vi "dashboard_vision_processing.vi"(11 "Image Ctl":refnum<vi>) -> ()   [LabVIEW 2011]
uses:
  dashboard_return_data.ctl
  2012vision/Camera State.ctl
  <vilib>/vision/NI_Vision_Development_Module.lvlib
panel:
  out "error out":errorcluster
  in  "Threshold Range":cluster{"Lower value":sgl, "Upper value":sgl}={"Lower value"=217.0, "Upper value"=255.0} {"Upper value" format="%.2f"; "Lower value" format="%.2f"}
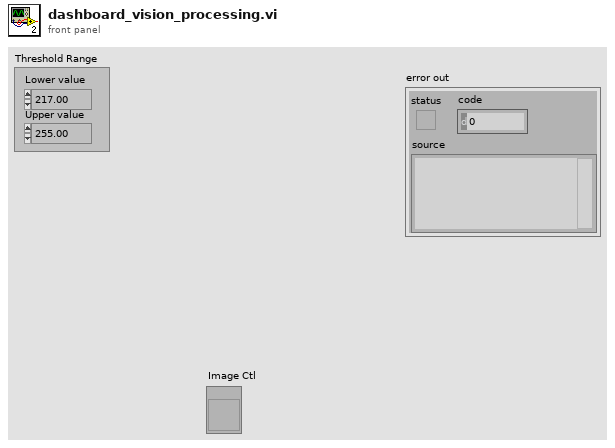
[diagram p1: front panel]
types:
  T1 = typedef "Image Type" = u32
  T2 = typedef "IMAQ Image.ctl" = refnum<image>
  T3 = typedef "dashboard_return_data.ctl" = cluster{"Targetting Output":cluster{"X Position":dbl, "Distance":dbl, "Camera State":T4}, "Camera Error Status":errorcluster, "packet send timestamp":u32, "img process timestamp":u32}
  T4 = typedef "Camera State.ctl" = enum16{"No Targets", "Low Confidence", "Medium Confidence", "High Confidence", "Camera Error"}
  T5 = enum32{"AutoM", "Close", "Dilate", "Erode", "Gradient", "Gradient in", "Gradient out", "HitMiss", "Open", "PClose", "POpen", "Thick", "Thin"}
  T6 = cluster{"Rect Coverage":dbl, "Aspect Ratio":dbl, "X Edge Strength":dbl, "Y Edge Strength":dbl}
  T7 = typedef "WPI_CameraImageSize.ctl" = enum16{"640x480", "320x240", "160x120"}
  T8 = cluster{"fps dashboard":i32, "compression dashboard":i32, "img size dashboard":T7}
  T9 = cluster{cluster{"Left":dbl, "Top":dbl, "Right":dbl, "Bottom":dbl}, cluster{"Score":dbl, "Score":dbl, "X Score":dbl, "Y Score":dbl}, "Clipped Edge":cluster{"Left":bool, "Top":bool, "Right":bool, "Bottom":bool}}[]
  T10 = cluster{"X Position":dbl, "Distance":dbl, "Camera State":T4}
  T11 = typedef "Diamond Target Output.ctl" = cluster{"Position":cluster{"X":dbl, "Y":dbl, "Distance":dbl}, "Est. Position":T12, "Target Confidence":T13}
  T12 = typedef "Rectangle Position.ctl" = enum16{"Unknown", "Top", "Right", "Left", "Bottom"}
  T13 = typedef "Target Confidence.ctl" = enum16{"Good", "Good-Clipped Y", "Marginal-Clipped X"}
  T14 = typedef "Line.ctl" = cluster{"First Point":cluster{"X":dbl, "Y":dbl, "Index":dbl}, "Second Point":cluster{"X":dbl, "Y":dbl, "Index":dbl}, "theta":dbl, "Direction":T15, "Line Confidence":T16}
  T15 = typedef "Direction.ctl" = enum16{"Rt", "Rt-Up", "Up", "Lt-Up", "Lt", "Lt-Dn", "Dn", "Rt-Dn", "Unknown"}
  T16 = typedef "Line Confidence.ctl" = enum16{"Good", "Bad"}
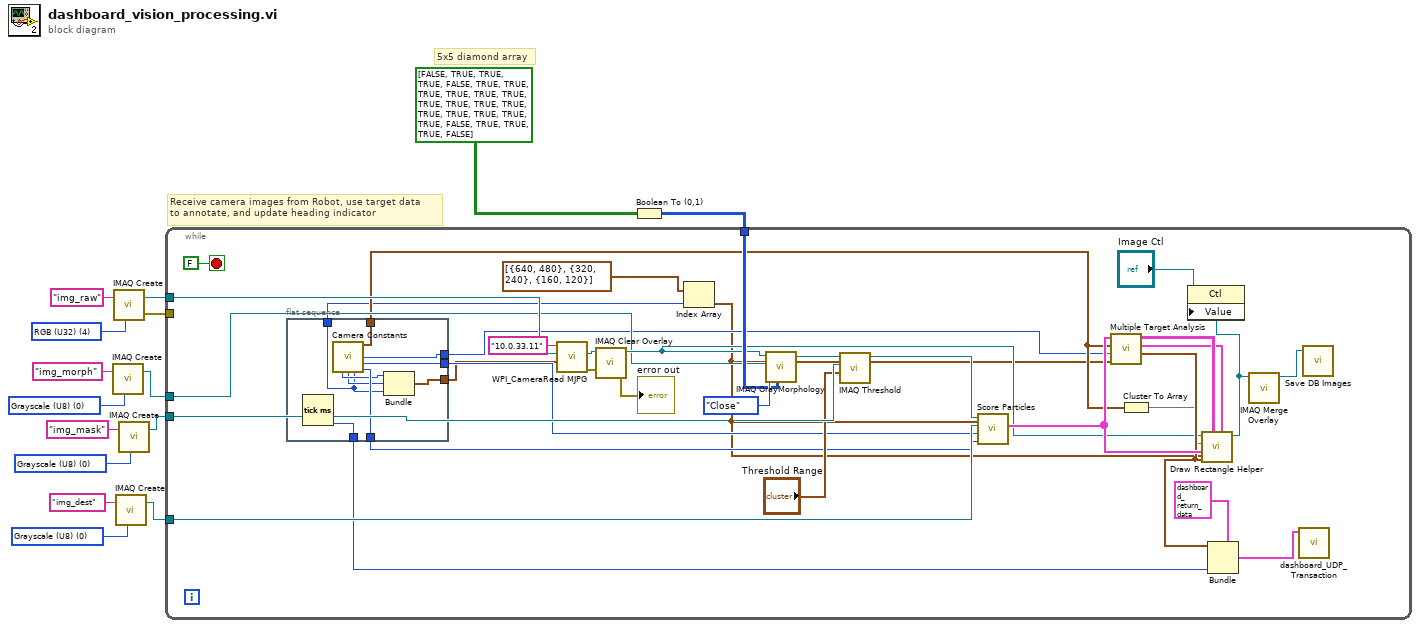
[diagram p0: block diagram]
diagram:
  w4 = T1 0 items=["Grayscale (U8)", "Grayscale (I16)", "Grayscale (SGL)", "Complex (CSG)", "RGB (U32)", "HSL (U32)", "RGB (U64)"] ("Image Type")
  w14 = T1 0 items=["Grayscale (U8)", "Grayscale (I16)", "Grayscale (SGL)", "Complex (CSG)", "RGB (U32)", "HSL (U32)", "RGB (U64)"] ("Image Type")
  w11 = T1 0 items=["Grayscale (U8)", "Grayscale (I16)", "Grayscale (SGL)", "Complex (CSG)", "RGB (U32)", "HSL (U32)", "RGB (U64)"] ("Image Type")
  w7 = T1 4 items=["Grayscale (U8)", "Grayscale (I16)", "Grayscale (SGL)", "Complex (CSG)", "RGB (U32)", "HSL (U32)", "RGB (U64)"] ("Image Type")
  # "5x5 diamond array"
  # "Receive camera images from Robot, use target data\nto annotate, and update heading indicator"
  n1 = call "IMAQ Create"("Image Name"="img_morph", "Image Type"=w11) -> ("New Image"=w13:T2)  [unwired: 2 in, 2 out]
  n2 = call "IMAQ Create"("Image Name"="img_raw", "Image Type"=w7) -> ("New Image"=w9:T2, "error out"=w10:errorcluster)  [unwired: 2 in, 1 out]
  n3 = call "IMAQ Create"("Image Name"="img_dest", "Image Type"=w4) -> ("New Image"=w3:T2)  [unwired: 2 in, 2 out]
  n4 = call "IMAQ Create"("Image Name"="img_mask", "Image Type"=w14) -> ("New Image"=w6:T2)  [unwired: 2 in, 2 out]
  n5 = Boolean To (0,1)(Boolean=bool[][] [[FALSE, TRUE, TRUE, TRUE, FALSE], [TRUE, TRUE, TRUE, TRUE, TRUE], [TRUE, TRUE, TRUE, TRUE, TRUE], [TRUE, TRUE, TRUE, TRUE, TRUE], [FALSE, TRUE, TRUE, TRUE, FALSE]]) -> (0, 1=w2:i16[][])
  n6 = while {
    tunnel: w9 -> [w47]
    tunnel: w10 -> [_]
    tunnel: w13 -> [w25]
    tunnel: w2 -> [w28]
    tunnel: w6 -> [w42]
    tunnel: w3 -> [w39]
    stop <- FALSE stop-if-true
    n7 = flat-sequence {
      tunnel: [w57] -> w29
      tunnel: [w56] -> w24
      tunnel: [w55] -> w23
      tunnel: [w54] -> w22
      tunnel: [w53] -> w21
      tunnel: [w50] -> w20
      tunnel: [w49] -> w18
      frame #0 {
        n8 = Tick Count (ms)() -> (millisecond timer value=w57:u32)
        n9 = call "Camera Constants.vi"() -> ("score limits"=w56:T6, "cam type"=w50:enum16{"206", "1011"}, "particle count limit"=w55:i32, "fps dashboard"=w52:i32, "compression dashboard"=w51:i32, "img size dashboard"=w49:T7, "area size limit"=w54:i32)  [unwired: 5 in, 4 out]
        n10 = Bundle("fps dashboard"=w52, "compression dashboard"=w51, "img size dashboard"=w49) -> (w53:T8)  [unwired: 1 in]
      }
    }
    n11 = call <vilib>:"WPI_CameraRead MJPG.vi"("Camera Settings"=w21, "Image"=w47, "address"="10.0.33.11") -> ("error out"=→"error out":errorcluster, "Image Out"=w46:T2)  [unwired: 7 in]
    n12 = call "IMAQ Clear Overlay"("Image"=w46) -> ("Image Out"=w26:T2)  [unwired: 2 in, 8 out]
    n13 = Index Array(array=cluster{i32, i32}[] [{640, 480}, {320, 240}, {160, 120}], index=w18) -> (element=w17:cluster{i32, i32})
    n14 = call "IMAQ GrayMorphology"("Structuring Element"=w28, "Operation"=T5."Close", "Image Dst"=w25, "Image Src"=w26) -> ("Image Dst Out"=w43:T2)  [unwired: 6 in, 1 out]
    n15 = call "IMAQ Threshold"("Range"="Threshold Range", "Image Dst"=w42, "Image Src"=w43) -> ("Image Dst Out"=w40:T2)  [unwired: 7 in, 1 out]
    n16 = call "Score Particles.vi"("Image Size"=w17, "Area Size Limit"=w22, "Particle Count Limit"=w23, "Image Dst"=w39, "Image Refnum in"=w40) -> ("Targets"=w36:T9)  [unwired: 5 in, 1 out]
    n17 = call "Multiple Target Analysis.vi"("Image Size"=w17, "Camera Type"=w20, "Score Limits"=w24, "Targets"=w36) -> ("Targetting Output"=w30:T10, "Diamond Targets"=w37:T11[], "Lines"=w38:T14[][])  [unwired: 5 in]
    n18 = Cluster To Array(cluster=w24) -> (array=w27:dbl[])
    n19 = call "Draw Rectangle Helper.vi"("Diamond Targets"=w37, "Image Size"=w17, "Lines"=w38, "Targetting Output"=w30, "Targets"=w36, "Score Limits"=w27, "Refnum in"=w26) -> ("Refnum out"=w33:T2)  [unwired: 4 in]
    n20 = property on="Property Node" class="Ctl"(reference="Image Ctl", "Value"=w33) -> ()  [unwired: 1 in, 2 out]
    n21 = Bundle(cluster=T3 {"Targetting Output"={"X Position"=0.0, "Distance"=0.0, "Camera State"=enum."No Targets"}, "Camera Error Status"={"status"=FALSE, "code"=0, "source"=""}, "packet send timestamp"=0, "img process timestamp"=0} ("Dashboard Return Data"), "Targetting Output"=w30, "img process timestamp"=w29) -> (w31:T3)  [unwired: 2 in]
    n22 = call "IMAQ Merge Overlay"("Image Src"=w33) -> ("Image Dst Out"=w34:T2)  [unwired: 9 in, 1 out]
    n23 = call "dashboard_UDP_Transaction.vi"("Dashboard Return Data"=w31) -> ()  [unwired: 11 in]
    n24 = call "Save DB Images.vi"("Image"=w34) -> ()  [unwired: 2 in, 1 out]
  }
